vi "PCO_GetBitAlignment.vi"(8 "error in (no error)":errorcluster, 11 "Handle":u64) -> (0 "error out":errorcluster, 3 "Handle Out":u64, 5 "return type":u32 format="%x", 10 "wBitAlignment":enum16{"MSB", "LSB"}(ring))   [LabVIEW 2011]
uses:
  SC2_Cam64.dll
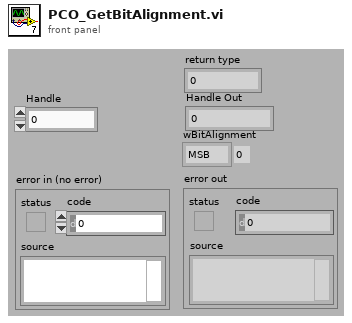
[diagram p1: front panel]
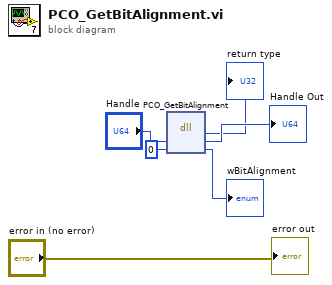
[diagram p0: block diagram]
diagram:
  n1 = dll-call lib="C:/Program Files/colibri/Drivers/PCO.Camera/SC2_Cam*.*" fn="PCO_GetBitAlignment"("Handle"="Handle", "wBitAlignment"=u16 0) -> ("return type"=→"return type":u32, "Handle"=→"Handle Out":u64, "wBitAlignment"=→"wBitAlignment":u16)  [unwired: 3 in, 2 out]
  "error out" <- "error in (no error)"
